vi "ExerciseE1.1.vi"() -> ()   [LabVIEW 2018]
panel:
  out "Numeric":i32
  out "Waveform Graph":dbl[](graph)
  out "Waveform Chart":dbl(graph)
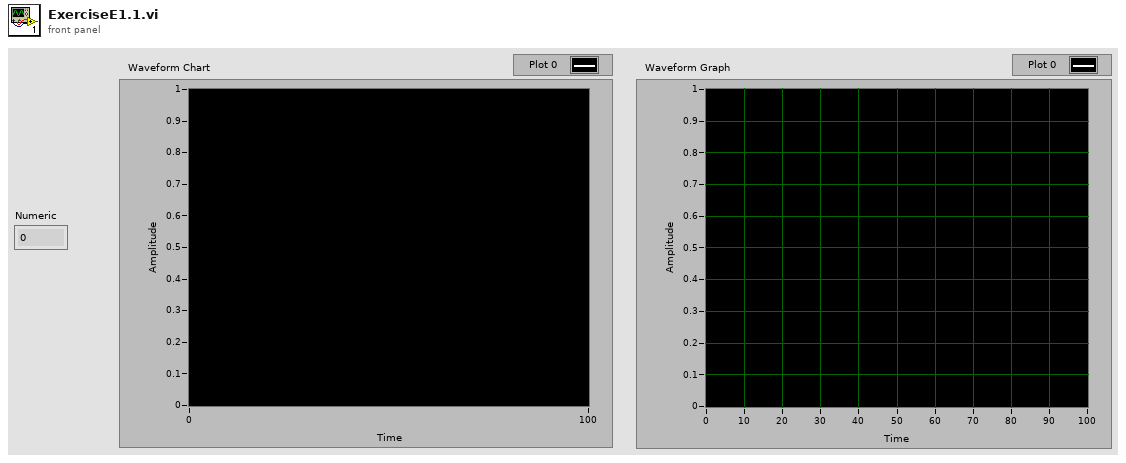
[diagram p1: front panel]
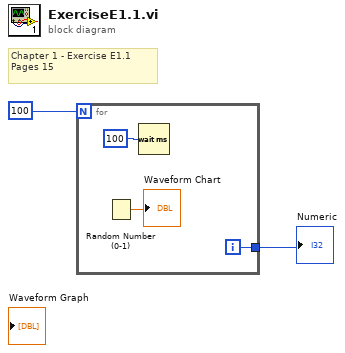
[diagram p0: block diagram]
diagram:
  # "Chapter 1 - Exercise E1.1\nPages 15"
  n1 = for {
    N: 100 -> [_]
    tunnel: [w3] -> w1
    i -> [w3]
    n2 = Random Number (0-1)() -> (number: 0 to 1=→"Waveform Chart":dbl)
    n3 = Wait (ms)(milliseconds to wait=u32 100) -> ()  [unwired: 1 out]
  }
  "Numeric" <- w1
